vi "Set_curr.vi"(8 "error in (no error)":errorcluster, 10 "Current":dbl, 11 "VISA resource in":refnum<visa-resource-name>) -> (0 "error out":errorcluster, 3 "VISA resource out":refnum<visa-resource-name>)   [LabVIEW 2014, in "B&K Precision 9120 series.lvclass"]
uses:
  B&K Precision 9120 series.lvclass
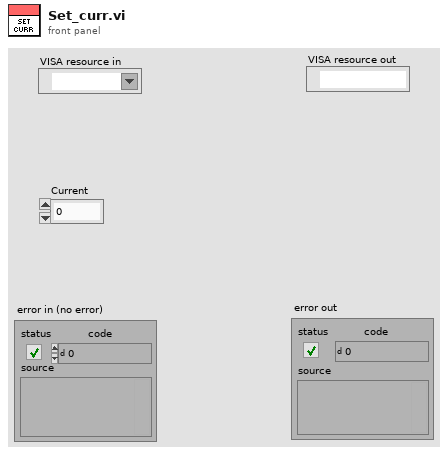
[diagram p1: front panel]
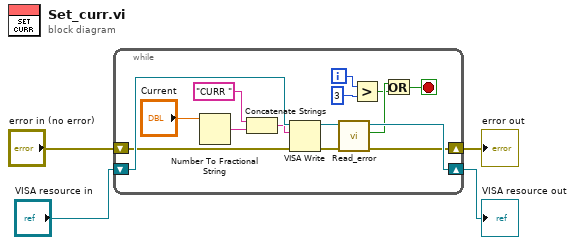
[diagram p0: block diagram]
diagram:
  n1 = while {
    shift-right: [w11] -> w2
    shift-left: "VISA resource in" -> [w19]
    shift-right: [w10] -> w1
    shift-left: "error in (no error)" -> [w18]
    i -> [w6]
    stop <- w9 stop-if-true
    n2 = Number To Fractional String(number="Current") -> (F-format string=w15:string)  [unwired: 3 in]
    n3 = Concatenate Strings("CURR " ("write buffer"), w15) -> (w17:string)
    n4 = VISA Write(VISA resource name=w19, write buffer=w17, error in (no error)=w18) -> (VISA resource name out=w13:refnum<visa-resource-name>, error out=w12:errorcluster)  [unwired: 1 out]
    n5 = call "Read_error.vi"("error in (no error)"=w12, "VISA resource in"=w13) -> ("error out"=w10:errorcluster, "OK"=w8:bool, "VISA resource out"=w11:refnum<visa-resource-name>)  [unwired: 7 in]
    n6 = Greater?(x=w6, y=3) -> (0:w7:bool)
    n7 = Or(x=w8, y=w7) -> (x .or. y?=w9:bool)
  }
  "VISA resource out" <- w2
  "error out" <- w1
